vi "Use_Key_Pad_Numerics.vi"(8 "error in (no error)":errorcluster, 10 "Key Pad":i32, 11 "Display in":string) -> (0 "error out":errorcluster, 2 "Elaspsed Time":dbl, 3 "Display out":string)   [LabVIEW 2026]
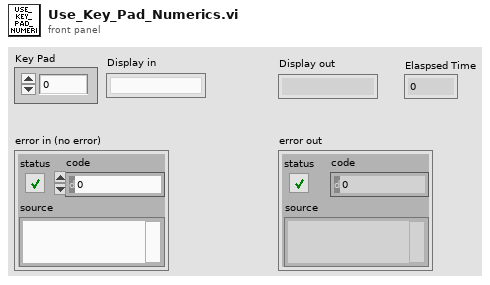
[diagram p1: front panel]
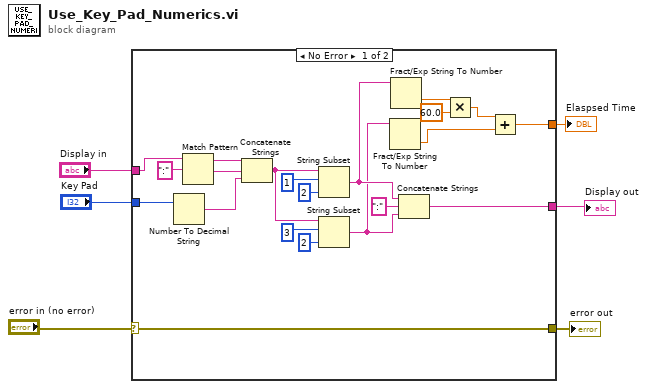
[diagram p0: block diagram]
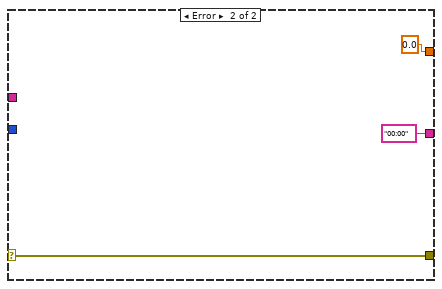
[diagram p2: hidden frame]
diagram:
  n1 = case shown="No Error" "error in (no error)" {
    selector: "error in (no error)" -> [w27 w30]
    tunnel: [w27 w30] -> w5
    tunnel: "Key Pad" -> [w23 _]
    tunnel: "Display in" -> [w26 _]
    tunnel: [w17 "00:00"] -> w2
    tunnel: [w9 0.0] -> w1
    frame No Error {
      n2 = Number To Decimal String(number=w23) -> (decimal integer string=w12:string)  [unwired: 1 in]
      n3 = Match Pattern(string=w26, regular expression=":") -> (before substring=w15:string, after substring=w24:string)  [unwired: 1 in, 2 out]
      n4 = Concatenate Strings(w15, w24, w12) -> (w16:string)
      n5 = String Subset(string=w16, offset (0)=1, length (rest)=2 ("length (rest)")) -> (substring=w8:string)
      n6 = String Subset(string=w16, offset (0)=3, length (rest)=2 ("length (rest)")) -> (substring=w7:string)
      n7 = Fract/Exp String To Number(string=w7) -> (number=w10:dbl)  [unwired: 3 in, 1 out]
      n8 = Fract/Exp String To Number(string=w8) -> (number=w14:dbl)  [unwired: 3 in, 1 out]
      n9 = Concatenate Strings(w8, ":" ("regular expression"), w7) -> (w17:string)
      n10 = Multiply(x=w14, y=60.0) -> (x*y=w11:dbl)
      n11 = Add(x=w11, y=w10) -> (x+y=w9:dbl)
    }
    frame Error {
    }
  }
  "Display out" <- w2
  "error out" <- w5
  "Elaspsed Time" <- w1
